vi "MC - Test Date String.vi"(0 "date string":string) -> (1 "valid date":bool, 2 "the string is \"date\"":bool)   [LabVIEW 2015]
panel:
  in  "date time rec":T1
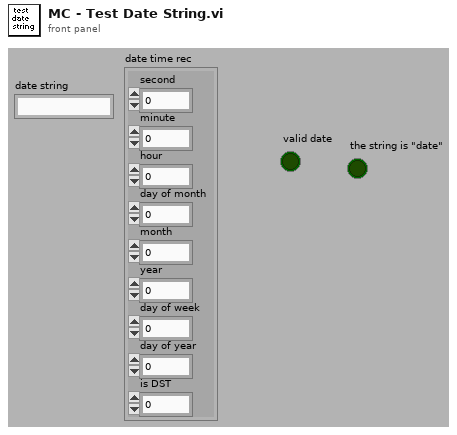
[diagram p1: front panel]
types:
  T1 = cluster{"second":i32, "minute":i32, "hour":i32, "day of month":i32, "month":i32, "year":i32, "day of week":i32, "day of year":i32, "is DST":i32}
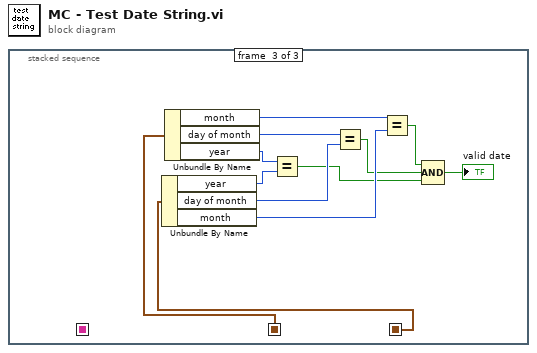
[diagram p0: block diagram]
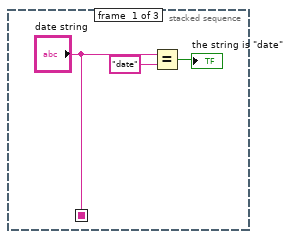
[diagram p2: hidden frame]
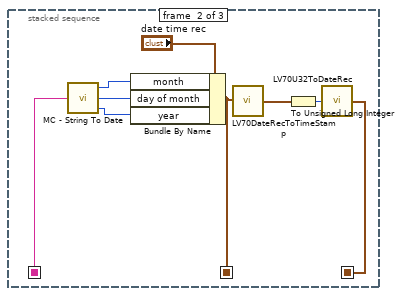
[diagram p3: hidden frame]
diagram:
  n1 = stacked-sequence {
    seq-local: [_ w9 _] -> [_ _ w24]
    seq-local: [_ w8 _] -> [_ _ w23]
    seq-local: ["date string" _ _] -> [_ w4 _]
    frame #0 {
      n2 = Equal?(x="date string", y="date") -> (x = y?=→"the string is \"date\"":bool)
    }
    frame #1 {
      n3 = call "MC - String To Date.vi"("String Date"=w4) -> ("Month"=w11:u32, "Day"=w10:u32, "Year"=w7:u32)
      n4 = Bundle By Name(cluster="date time rec", "month"=w11, "day of month"=w10, "year"=w7) -> (w9:T1)
      n5 = call <vilib>:"LV70DateRecToTimeStamp.vi"("date time rec"=w9) -> ("Time Stamp"=w5:timestamp)
      n6 = To Unsigned Long Integer(number=w5) -> (unsigned 32bit integer=w6:u32)
      n7 = call <vilib>:"LV70U32ToDateRec.vi"("Time"=w6) -> ("date time rec"=w8:T1)
    }
    frame #2 {
      n8 = Unbundle By Name(w23) -> ("year"=w21:i32, "day of month"=w19:i32, "month"=w17:i32)
      n9 = Unbundle By Name(w24) -> ("month"=w18:i32, "day of month"=w20:i32, "year"=w22:i32)
      n10 = Equal?(x=w22, y=w21) -> (x = y?=w14:bool)
      n11 = Equal?(x=w20, y=w19) -> (x = y?=w15:bool)
      n12 = Equal?(x=w18, y=w17) -> (x = y?=w16:bool)
      n13 = Compound Arithmetic op=AND(w16, w15, w14) -> (→"valid date":bool)
    }
  }
